vi "Diagnostics-Add Noise.vi"(0 "Signal":dbl[](array[numeric]), 9 "Noise RMS":dbl=0.5) -> (4 "Signal + Noise":dbl[](array[numeric]))   [LabVIEW 2015]
uses:
  <vilib>/Analysis/NI_AALBase.lvlib
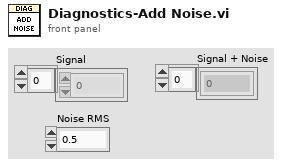
[diagram p1: front panel]
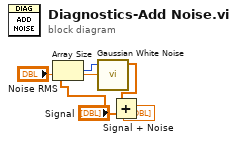
[diagram p0: block diagram]
diagram:
  n1 = Array Size(array="Signal") -> (size(s)=w3:i32)
  n2 = call <vilib>:"Gaussian White Noise.vi"("standard deviation"="Noise RMS", "samples"=w3) -> ("Gaussian noise pattern"=w4:dbl[])  [unwired: 8 in, 1 out]
  n3 = Add(x=w4, y="Signal") -> (x+y=→"Signal + Noise":dbl[])
